vi "oscilloscope.vi"() -> ()   [LabVIEW 2011]
panel:
  in  "filename":string="C:\\Users\\jhkoivis\\Documents\\programming\\dvelib\\alpha\\labviewTraining\\01_basics\\01_basics"
  out "Waveform Chart":dbl(graph)
  in  "InitialValue":dbl
  in  "Stop":bool
  out "FrequencyOut":dbl
  in  "Frequency":i16=2
  # "MY PROGRAM"
  # "make current\nvalue default"
  # "Exercise: Make your own program that writes floats. Each float to its own line.\nHint: Scan Value, concatenate strings"
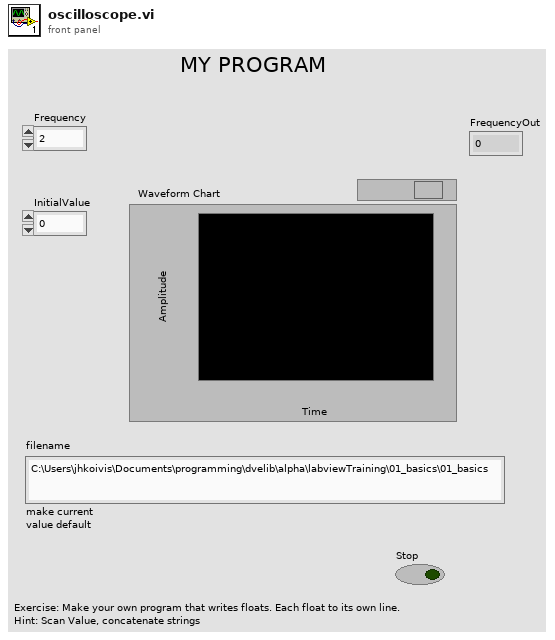
[diagram p1: front panel]
types:
  T1 = enum16{"open", "replace", "create", "open or create", "replace or create", "replace or create with confirmation"}
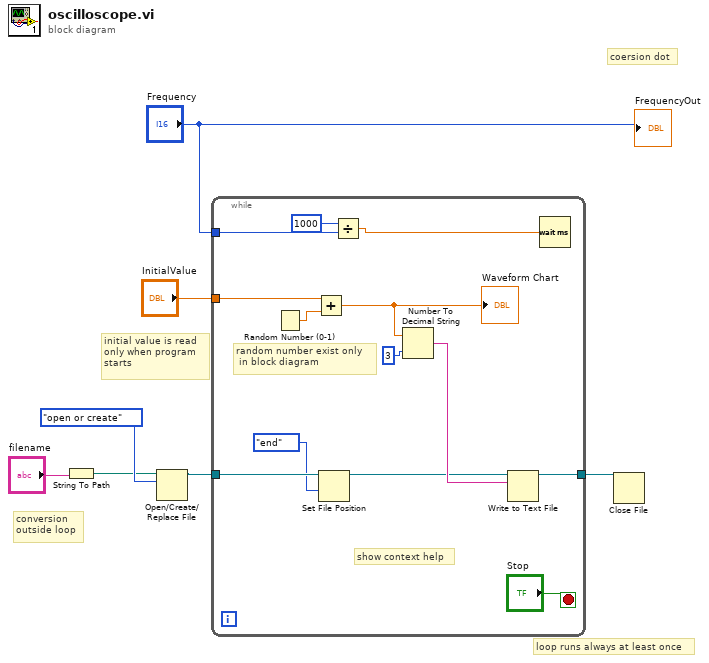
[diagram p0: block diagram]
diagram:
  # "conversion\noutside loop"
  # "initial value is read\nonly when program\nstarts"
  # "loop runs always at least once"
  # "coersion dot"
  n1 = String To Path(string="filename") -> (path=w3:path)
  n2 = Open/Create/Replace File(file path (use dialog)=w3, operation (0:open)=T1."open or create") -> (refnum out=w2:refnum<file>)  [unwired: 4 in, 2 out]
  n3 = while {
    tunnel: "Frequency" -> [w20]
    tunnel: "InitialValue" -> [w16]
    tunnel: w2 -> [w11]
    tunnel: [w8] -> w1
    stop <- "Stop" stop-if-true
    # "show context help"
    # "random number exist only\n in block diagram"
    n4 = Random Number (0-1)() -> (number: 0 to 1=w15:dbl)
    n5 = Add(x=w16, y=w15) -> (x+y=w14:dbl)
    "Waveform Chart" <- w14
    n6 = Set File Position(refnum=w11, from (0:start)=enum16{"start", "end", "current"}."end") -> (refnum out=w10:refnum<file>)  [unwired: 2 in, 1 out]
    n7 = Divide(x=i16 1000, y=w20) -> (x/y=w18:dbl)
    n8 = Number To Decimal String(number=w14, width (-)=i16 3) -> (decimal integer string=w13:string)
    n9 = Write to Text File(file (use dialog)=w10, text=w13) -> (refnum out=w8:refnum<file>)  [unwired: 2 in, 2 out]
    n10 = Wait (ms)(milliseconds to wait=w18) -> ()  [unwired: 1 out]
  }
  n11 = Close File(refnum=w1) -> ()  [unwired: 1 in, 2 out]
  "FrequencyOut" <- "Frequency"
